vi "LTVDiffDriveCtrl_New.vi"(6 "dT":dbl=0.02, 8 "Relms":T2=[[0.0], [0.0]], 9 "Qelms":T2=[[0.0], [0.0], [0.0], [0.0], [0.0]], 10 "TrackWidth":dbl=0.7, 11 "Plant":T1) -> (0 "Error":bool, 3 "DiffDriveCtrl":T3)   [LabVIEW 2019, in "Trajectory_Library.lvlib"]
doc: "Calculate the accelerationlimited differential drive output voltages \nInputs:\n - DiffDriveAccelLimit -- Data cluster\n\nOutputs:\n - Error -- If TRUE, an error occured."
uses:
  Trajectory_Library.lvlib
  LTV_DIFF_DRIVE_CTRL.ctl
  FUNCTION_GENERATOR_MATRIX.ctl
  <vilib>/Analysis/Matrix/Datatypes/RealMatrix.ctl
  LINEAR_SYSTEM.ctl
  LTV_DIFF_DRIVE_CTRL_STATE_ENUM.ctl
  <vilib>/Analysis/baseanly.llb/Real A x B.vi
  MatBuilder_Create.vi
  MatrixHelper_CoerceSize.vi
  <vilib>/Analysis/7linalg.llb/Solve Linear Equations (multiple right hand).vi
  <vilib>/Analysis/Matrix/Numeric/Multiply/Multiply - RM,R.vi
  <vilib>/gmath/interp.llb/Search Ordered Table.vi
  <vilib>/Analysis/Matrix/NI_Matrix.lvlib
  <vilib>/Analysis/NI_AALPro.lvlib
  <vilib>/Analysis/NI_AALBase.lvlib
panel:
  # "<States,States>"
  # "<States,Inputs>"
  # "<Outputs,States>"
  # "<Outputs,Inputs>"
  # "< 5, 1 >"
  # "< 5, 1 >"
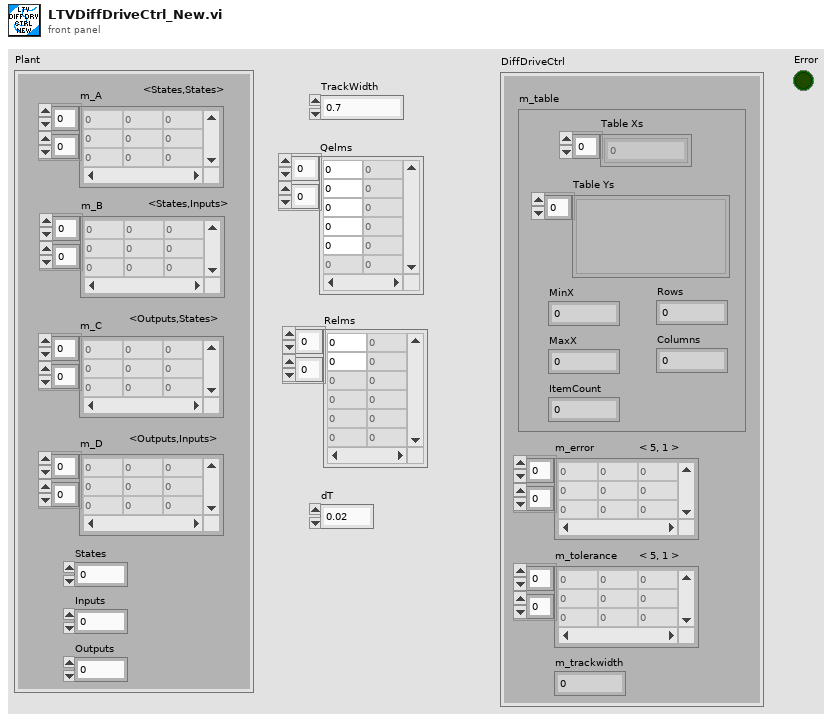
[diagram p1: front panel]
types:
  T1 = typedef "Trajectory_Library.lvlib/LINEAR_SYSTEM.ctl" = cluster{"m_A":T2, "m_B":T2, "m_C":T2, "m_D":T2, "States":i32, "Inputs":i32, "Outputs":i32}
  T2 = typedef "NI_Matrix.lvlib/RealMatrix.ctl" = dbl[][]
  T3 = typedef "Trajectory_Library.lvlib/LTV_DIFF_DRIVE_CTRL.ctl" = cluster{"m_table":T4, "m_error":T2, "m_tolerance":T2, "m_trackwidth":dbl}
  T4 = typedef "Trajectory_Library.lvlib/FUNCTION_GENERATOR_MATRIX.ctl" = cluster{"Table Xs":dbl[], "Table Ys":variant[], "MinX":dbl, "MaxX":dbl, "ItemCount":i32, "Rows":i32, "Columns":i32}
  T5 = typedef "Trajectory_Library.lvlib/LTV_DIFF_DRIVE_CTRL_STATE_ENUM.ctl" = enum16{"X_POS", "Y_POS", "HEADING", "LEFT_VEL", "RIGHT_VEL"}
  T6 = typedef "Trajectory_Library.lvlib/LINEAR_QUADRATIC_REGULATOR.ctl" = cluster{"m_r":T2, "m_U":T2, "m_K":T2, "States":i32, "Inputs":i32}
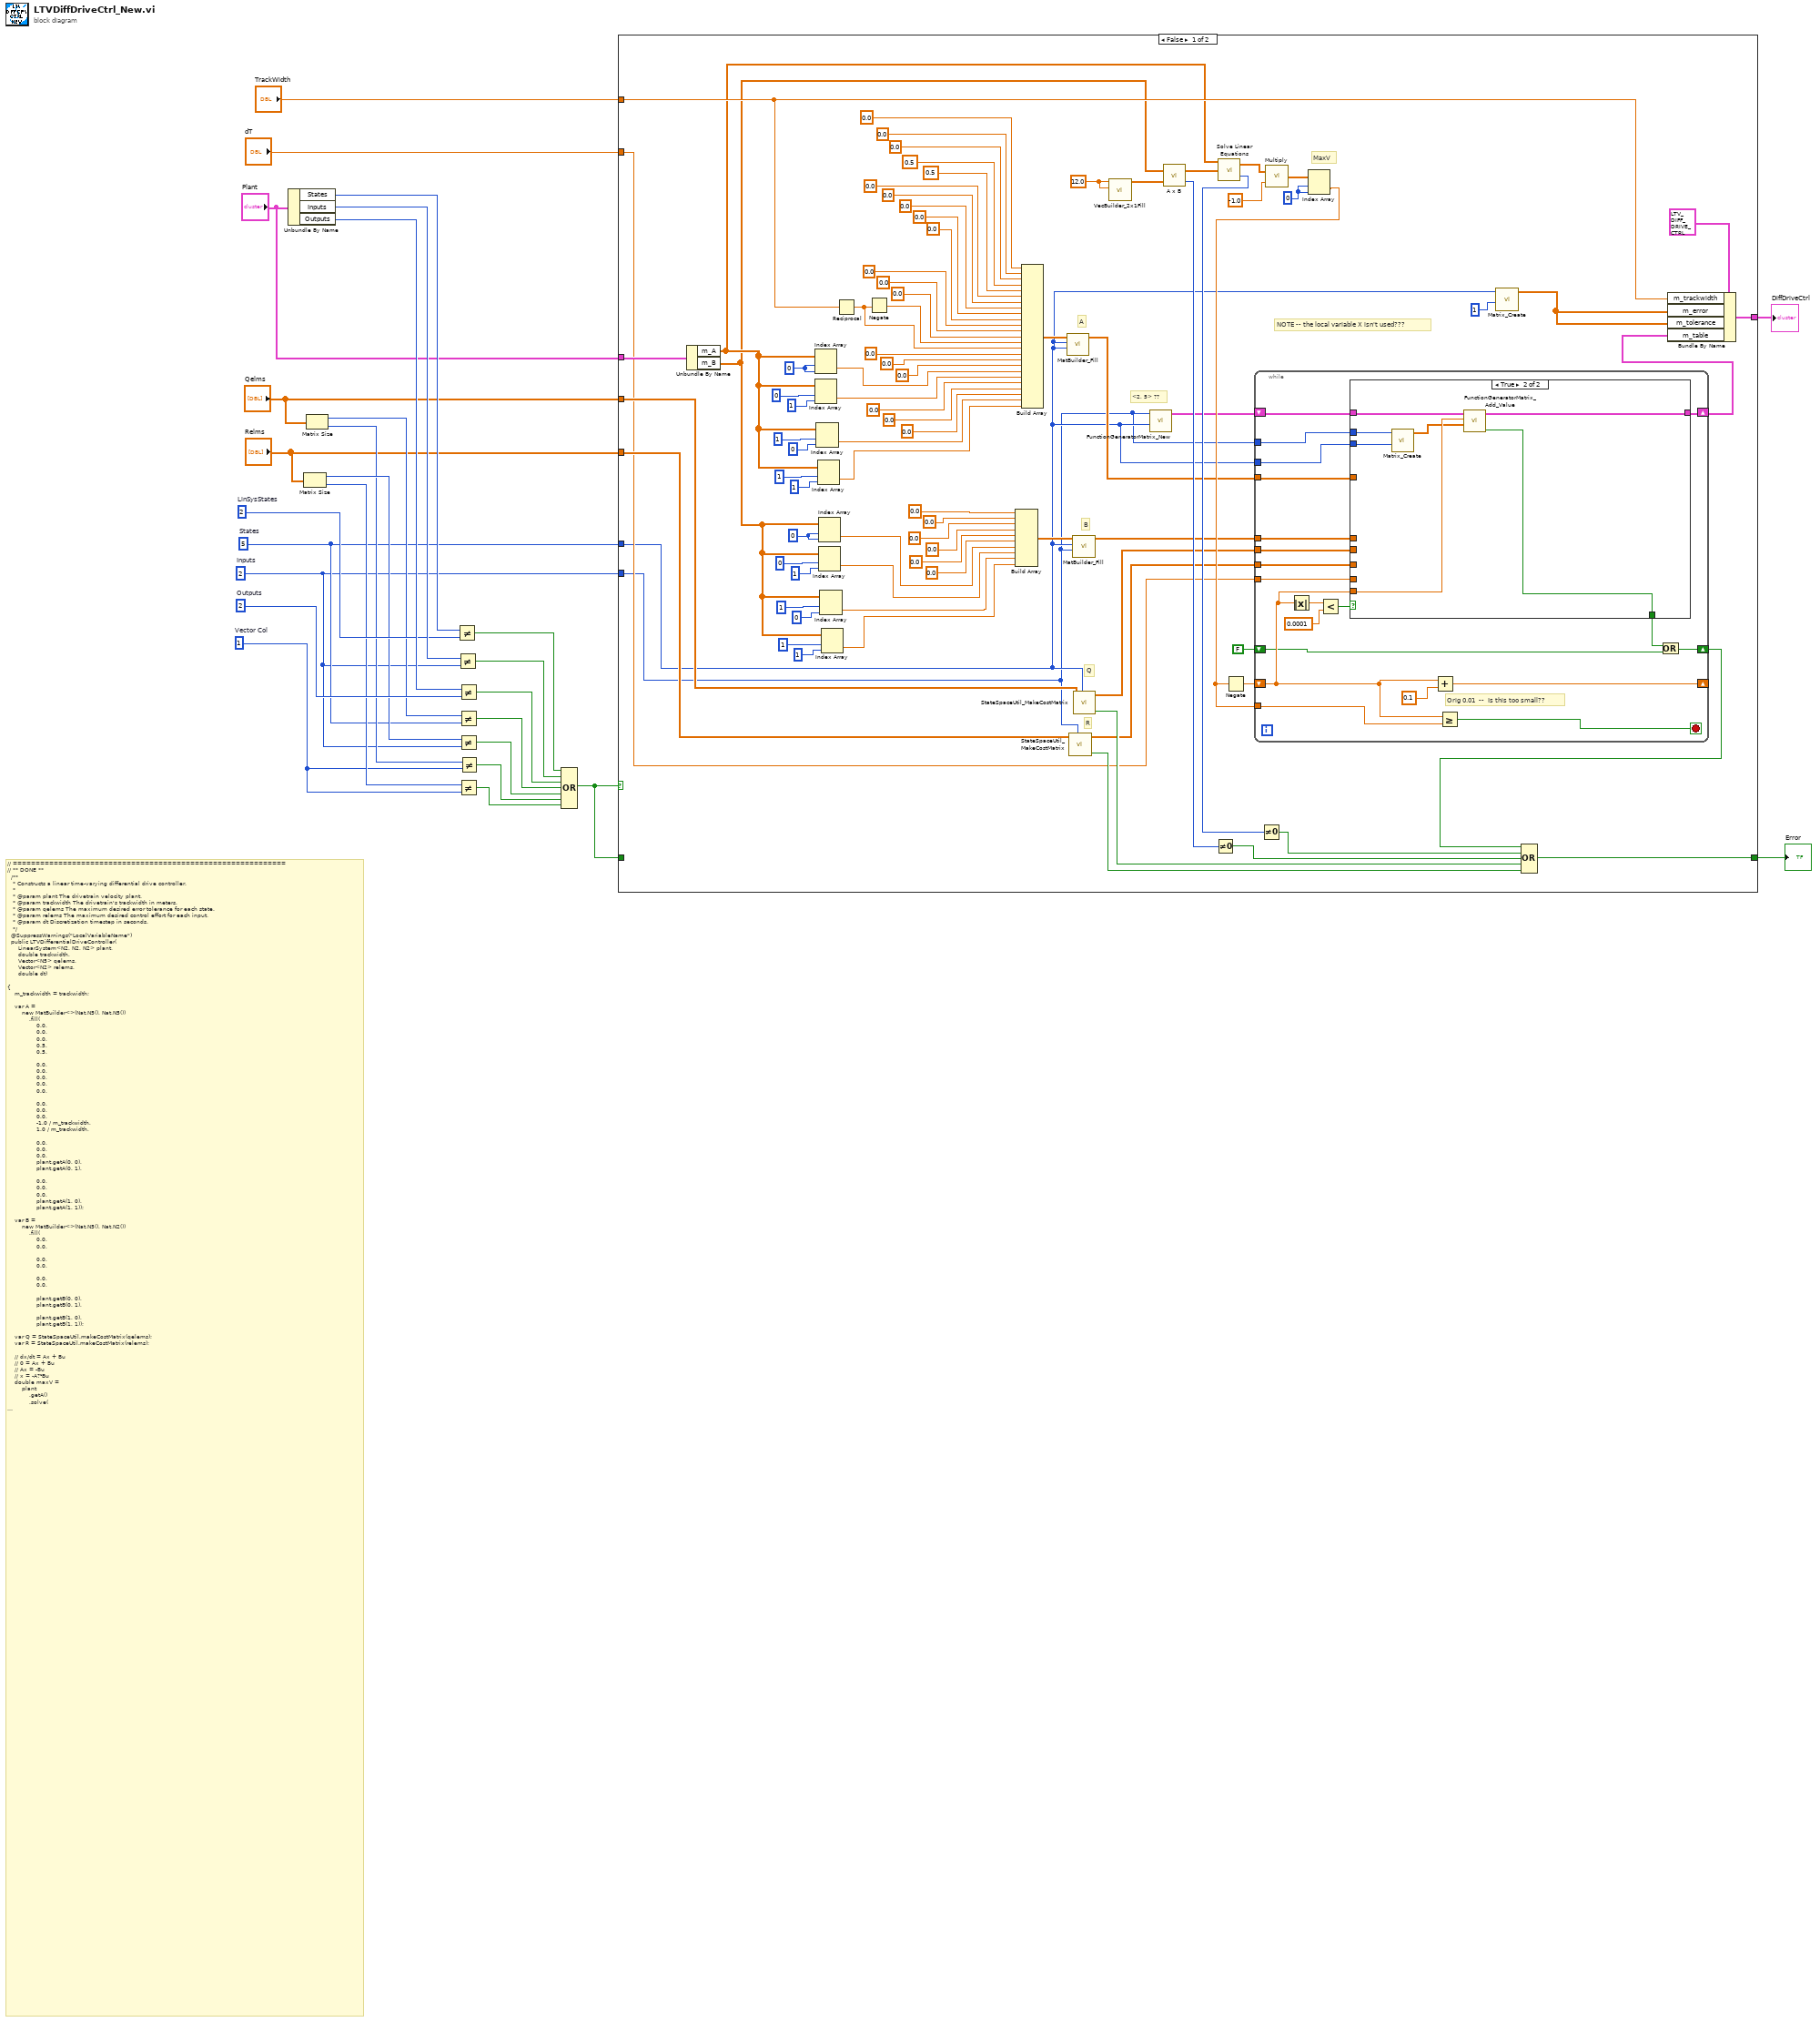
[diagram p0: block diagram]
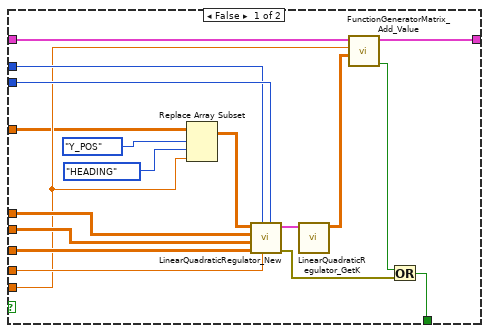
[diagram p2: hidden frame]
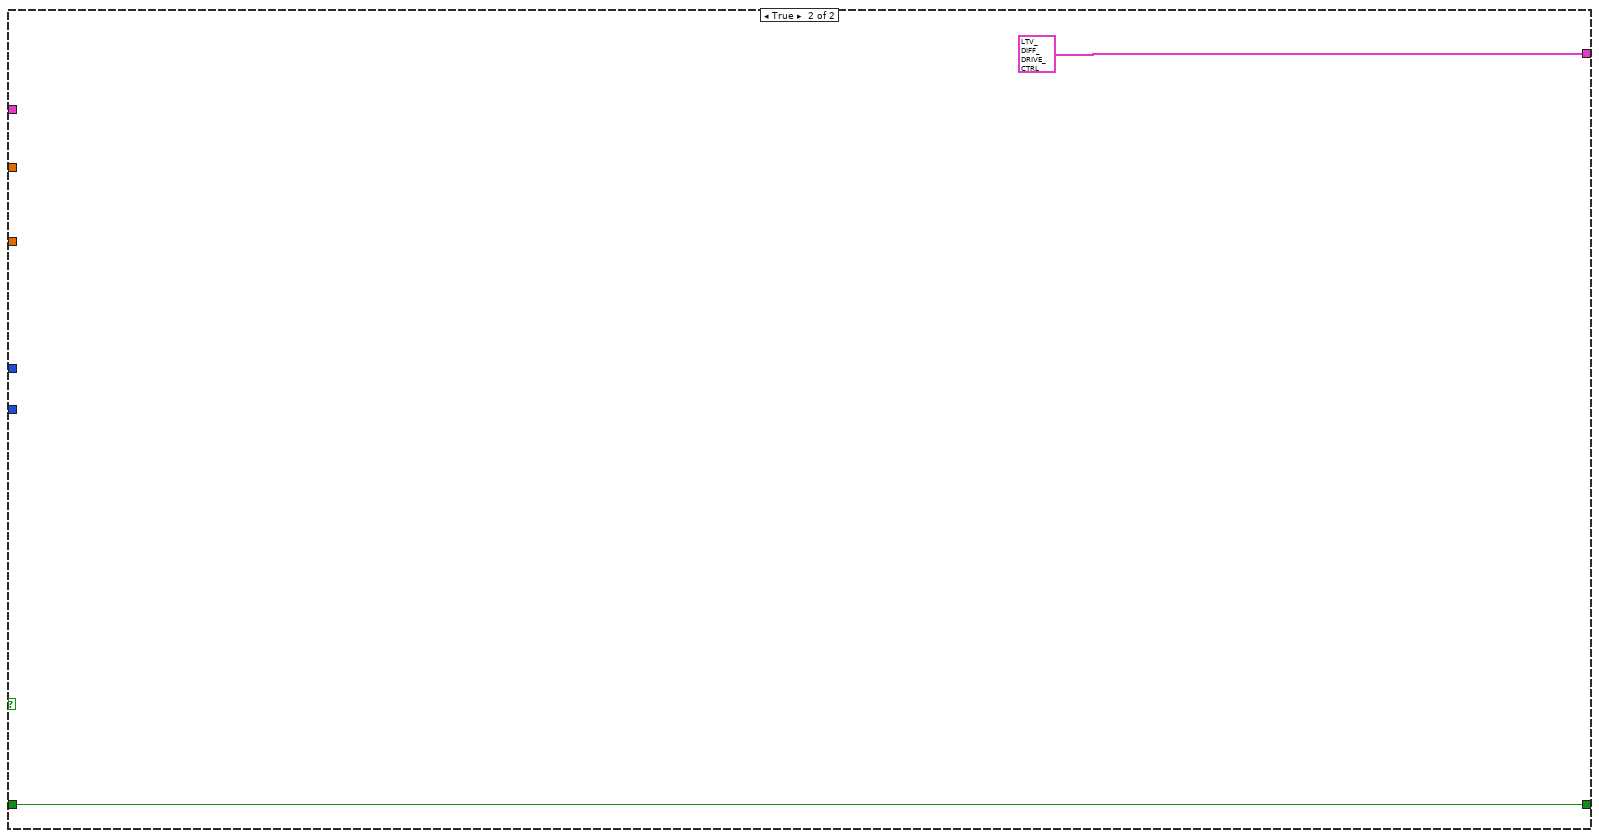
[diagram p3: hidden frame]
diagram:
  w18 = 1  # Vector Col
  w23 = 2  # Outputs
  w4 = 5  # States
  w24 = 2  # LinSysStates
  w1 = 2  # Inputs
  # "// ============================================================\n// ** DONE **\n  /**\n   * Constructs a linear time-varying differential drive controller.\n   *\n   * @param plant The drivetrain velocity plant.\n   * @param trackwidth The drivetrain's trackwidth in meters.\n   * @param qelems The maximum desired error tolerance for each state.\n   * @param relems The maximum desired control effort for each input.\n   * @param dt Discretization timestep in seconds.\n   */\n  @SuppressWarnings(\"LocalVariableName\")\n  public LTVDifferentialDriveController(\n      LinearSystem<N2, N2, N2> plant,\n      double trackwidth,\n      Vector<N5> qelems,\n      Vector<N2> relems,\n      double dt) \n\n{\n    m_trackwidth = trackwidth;\n\n    var A =\n        new MatBuilder<>(Nat.N5(), Nat.N5())\n            .fill(\n                0.0,\n                0.0,\n                0.0,\n                0.5,\n                0.5,\n\n                0.0,\n                0.0,\n                0.0,\n                0.0,\n                0.0,\n\n                0.0,\n                0.0,\n                0.0,\n                -1.0 / m_trackwidth,\n                1.0 / m_trackwidth,\n\n                0.0,\n                0.0,\n                0.0,\n                plant.getA(0, 0),\n                plant.getA(0, 1),\n\n                0.0,\n                0.0,\n                0.0,\n                plant.getA(1, 0),\n                plant.getA(1, 1));\n\n    var B =\n        new MatBuilder<>(Nat.N5(), Nat.N2())\n            .fill(\n                0.0,\n                0.0,\n\n                0.0,\n                0.0,\n\n                0.0,\n                0.0,\n\n                plant.getB(0, 0),\n                plant.getB(0, 1),\n\n                plant.getB(1, 0),\n                plant.getB(1, 1));\n\n    var Q = StateSpaceUtil.makeCostMatrix(qelems);\n    var R = StateSpaceUtil.makeCostMatrix(relems);\n\n    // dx/dt = Ax + Bu\n    // 0 = Ax + Bu\n    // Ax = -Bu\n    // x = -A?¹Bu\n    double maxV =\n        plant\n            .getA()\n            .solve(\n\t\tplant.getB().times(\n\t\t\tnew MatBuilder<>(Nat.N2(), Nat.N1()).fill(12.0, 12.0)))\n            .times(-1.0)\n            .get(0, 0);\n\n    var x = new Matrix<>(Nat.N5(), Nat.N1());\n\n    for (double velocity = -maxV; velocity < maxV; velocity += 0.01) {\n\n      x.set(State.kLeftVelocity.value, 0, velocity);\n      x.set(State.kRightVelocity.value, 0, velocity);\n\n      // The DARE is ill-conditioned if the velocity is close to zero, so don't\n      // let the system stop.\n      if (Math.abs(velocity) < 1e-4) {\n        m_table.put(velocity, new Matrix<>(Nat.N2(), Nat.N5()));\n      } else {\n        A.set(State.kY.value, State.kHeading.value, velocity);\n        m_table.put(velocity, new LinearQuadraticRegulator<N5, N2, N5>(A, B, Q, R, dt).getK());\n      }\n    }\n  }"
  n1 = Unbundle By Name("Plant") -> ("States"=w27:i32, "Inputs"=w26:i32, "Outputs"=w25:i32)
  n2 = Matrix Size(0:"Relms") -> (1:w21:i32, 2:w19:i32)
  n3 = Matrix Size(0:"Qelms") -> (1:w22:i32, 2:w20:i32)
  n4 = Not Equal?(x=w27, y=w24) -> (x != y?=w17:bool)
  n5 = Not Equal?(x=w26, y=w1) -> (x != y?=w16:bool)
  n6 = Not Equal?(x=w25, y=w23) -> (x != y?=w15:bool)
  n7 = Not Equal?(x=w22, y=w4) -> (x != y?=w14:bool)
  n8 = Not Equal?(x=w21, y=w1) -> (x != y?=w13:bool)
  n9 = Not Equal?(x=w19, y=w18) -> (x != y?=w11:bool)
  n10 = Not Equal?(x=w20, y=w18) -> (x != y?=w12:bool)
  n11 = Compound Arithmetic op=OR(w17, w16, w15, w14, w13, w12, w11) -> (w8:bool)
  n12 = case shown="False" w8 {
    tunnel: [w114 T3 {"m_table"={"Table Xs"=[], "Table Ys"=[], "MinX"=0.0, "MaxX"=0.0, "ItemCount"=0, "Rows"=0, "Columns"=0}, "m_error"=[], "m_tolerance"=[], "m_trackwidth"=0.0} ("LTV_DIFF_DRIVE_CTRL")] -> w10
    tunnel: [w32 w161] -> w9
    tunnel: w8 -> [_ w161]
    tunnel: "TrackWidth" -> [w92 _]
    tunnel: "Relms" -> [w113 _]
    tunnel: "Qelms" -> [w112 _]
    tunnel: w4 -> [w31 _]
    tunnel: "Plant" -> [w89 _]
    tunnel: w1 -> [w28 _]
    tunnel: "dT" -> [w35 _]
    frame False {
      w45 = 0 ("index (row)")
      w57 = 12.0 ("R0")
      w70 = 0 ("index (row)")
      w87 = 0 ("index (row)")
      # "NOTE -- the local variable X isn't used???"
      # "<2, 5> ??"
      # "MaxV"
      # "R"
      # "Q"
      # "B"
      # "A"
      n13 = Unbundle By Name(w89) -> ("m_A"=w58:T2, "m_B"=w55:T2)
      n14 = Index Array(array=w58, index (row)=w87, index (col)=w87) -> (element=w88:dbl)
      n15 = Index Array(array=w58, index (row)=0, index (col)=1) -> (element=w86:dbl)
      n16 = Index Array(array=w58, index (row)=1, index (col)=0) -> (element=w79:dbl)
      n17 = Index Array(array=w58, index (row)=1, index (col)=1) -> (element=w78:dbl)
      n18 = Index Array(array=w55, index (row)=w70, index (col)=w70) -> (element=w63:dbl)
      n19 = Index Array(array=w55, index (row)=0, index (col)=1) -> (element=w62:dbl)
      n20 = Index Array(array=w55, index (row)=1, index (col)=0) -> (element=w61:dbl)
      n21 = Index Array(array=w55, index (row)=1, index (col)=1) -> (element=w60:dbl)
      n22 = Reciprocal(x=w92) -> (1/x=w90:dbl)
      n23 = Negate(x=w90) -> (-x=w91:dbl)
      n24 = Build Array(0.0 ("element"), 0.0 ("element"), 0.0 ("element"), 0.0 ("element"), 0.0 ("element"), 0.0 ("element"), w63, w62, w61, w60) -> (w59:dbl[])
      n25 = Build Array(0.0 ("element"), 0.0 ("element"), 0.0 ("element"), 0.5 ("element"), 0.5 ("element"), 0.0 ("element"), 0.0 ("element"), 0.0 ("element"), 0.0 ("element"), 0.0 ("element"), 0.0 ("element"), 0.0 ("element"), 0.0 ("element"), w91, w90, 0.0 ("element"), 0.0 ("element"), 0.0 ("element"), w88, w86, 0.0 ("element"), 0.0 ("element"), 0.0 ("element"), w79, w78) -> (w77:dbl[])
      n26 = call "MatBuilder_Fill.vi"("Columns"=w31, "Rows"=w31, "Value List"=w77) -> ("output matrix"=w39:T2)  [unwired: 8 in]
      n27 = call "StateSpaceUtil_MakeCostMatrix.vi"("Elements"=w28, "Costs"=w113) -> ("Sze Coerced"=w51:bool, "Costs Matrix"=w36:T2)  [unwired: 8 in]
      n28 = call "MatBuilder_Fill.vi"("Columns"=w28, "Rows"=w31, "Value List"=w59) -> ("output matrix"=w38:T2)  [unwired: 8 in]
      n29 = call "StateSpaceUtil_MakeCostMatrix.vi"("Elements"=w31, "Costs"=w112) -> ("Sze Coerced"=w50:bool, "Costs Matrix"=w37:T2)  [unwired: 8 in]
      n30 = call "VecBuilder_2x1Fill.vi"("R1"=w57, "R0"=w57) -> ("output matrix"=w54:T2)  [unwired: 9 in]
      n31 = call "FunctionGeneratorMatrix_New.vi"("Columns"=w31, "Rows"=w28) -> ("FUNCTION_GENERATOR_MATRIX"=w41:T4)  [unwired: 9 in]
      n32 = call-poly <vilib>:"A x B.vi"("B"=w54, "A"=w55) -> ("error"=w49:i32, "A x B"=w56:T2)
      n33 = Not Equal To 0?(x=w49) -> (x != 0?=w48:bool)
      n34 = call-poly <vilib>:"Solve Linear Equations.vi"("Known Matrix"=w56, "Input Matrix"=w58) -> ("error"=w47:i32, "Solution Matrix"=w52:T2)  [unwired: 1 in]
      n35 = Not Equal To 0?(x=w47) -> (x != 0?=w46:bool)
      n36 = call-poly <vilib>:"Multiply.vi"("Real Scalar c"=-1.0 ("y"), "Real Matrix A"=w52) -> ("A * c"=w44:T2)
      n37 = Index Array(array=w44, index (row)=w45, index (col)=w45) -> (element=w42:dbl)
      n38 = Negate(x=w42) -> (-x=w43:dbl)
      n39 = while {
        shift-right: [w132] -> _
        shift-left: w43 -> [w125]
        tunnel: w42 -> [w134]
        shift-right: [w124] -> w40
        shift-left: w41 -> [w128]
        tunnel: w28 -> [w127]
        tunnel: w31 -> [w126]
        tunnel: w39 -> [w119]
        tunnel: w38 -> [w120]
        tunnel: w37 -> [w121]
        tunnel: w36 -> [w122]
        tunnel: w35 -> [w123]
        shift-right: [w116] -> w33
        shift-left: FALSE -> [w118]
        stop <- w133 stop-if-true
        # "Orig 0.01  --  Is this too small??"
        n40 = Absolute Value(x=w125) -> (abs(x)=w131:dbl)
        n41 = Less?(x=w131, y=0.0001) -> (x < y?=w129:bool)
        n42 = case shown="True" w129 {
          tunnel: w128 -> [w152 w158]
          tunnel: w127 -> [w145 w160]
          tunnel: w126 -> [w146 w159]
          tunnel: w125 -> [w143 w157]
          tunnel: [w153 w155] -> w124
          tunnel: w123 -> [w151 _]
          tunnel: w122 -> [w150 _]
          tunnel: w121 -> [w149 _]
          tunnel: w120 -> [w144 _]
          tunnel: w119 -> [w142 _]
          tunnel: [w138 w154] -> w117
          frame False {
            n43 = Replace Array Subset(array=w142, new element=w143, index (row)=LTV_DIFF_DRIVE_CTRL_STATE_ENUM."Y_POS" ("LTV_DIFF_DRIVE_CTRL_STATE"), index (col)=LTV_DIFF_DRIVE_CTRL_STATE_ENUM."HEADING" ("LTV_DIFF_DRIVE_CTRL_STATE")) -> (w141:T2)
            n44 = call "LinearQuadraticRegulator_New.vi"("States"=w146, "dt_Seconds"=w151, "Inputs"=w145, "R"=w150, "Q"=w149, "B"=w144, "A"=w141) -> ("Error"=w139:errorcluster, "LinearQuadraticRegulator"=w148:T6)  [unwired: 3 in]
            n45 = call "LinearQuadraticRegulator_GetK.vi"("in LinearQuadraticRegulator"=w148) -> ("K"=w147:T2)  [unwired: 10 in]
            n46 = call "FunctionGeneratorMatrix_Add_Value.vi"("Y Value"=w147, "X Value"=w143, "in FUNC_GEN_MATRIX"=w152) -> ("Error"=w140:bool, "out FUNC_GEN_MATRIX"=w153:T4)  [unwired: 7 in]
            n47 = Or(x=w140, y=w139) -> (x .or. y?=w138:bool)
          }
          frame True {
            n48 = call "Matrix_Create.vi"("Columns"=w159, "Rows"=w160) -> ("output matrix"=w156:T2)  [unwired: 9 in]
            n49 = call "FunctionGeneratorMatrix_Add_Value.vi"("Y Value"=w156, "X Value"=w157, "in FUNC_GEN_MATRIX"=w158) -> ("Error"=w154:bool, "out FUNC_GEN_MATRIX"=w155:T4)  [unwired: 7 in]
          }
        }
        n50 = Add(x=w125, y=0.1) -> (x+y=w132:dbl)
        n51 = Greater Or Equal?(x=w125, y=w134) -> (x >= y?=w133:bool)
        n52 = Or(x=w117, y=w118) -> (x .or. y?=w116:bool)
      }
      n53 = call "Matrix_Create.vi"("Columns"=1, "Rows"=w31) -> ("output matrix"=w29:T2)  [unwired: 9 in]
      n54 = Compound Arithmetic op=OR(w33, w46, w48, w50, w51) -> (w32:bool)
      n55 = Bundle By Name(cluster=T3 {"m_table"={"Table Xs"=[], "Table Ys"=[], "MinX"=0.0, "MaxX"=0.0, "ItemCount"=0, "Rows"=0, "Columns"=0}, "m_error"=[], "m_tolerance"=[], "m_trackwidth"=0.0} ("LTV_DIFF_DRIVE_CTRL"), "m_trackwidth"=w92, "m_error"=w29, "m_tolerance"=w29, "m_table"=w40) -> (w114:T3)
    }
    frame True {
    }
  }
  "DiffDriveCtrl" <- w10
  "Error" <- w9
